vi "Insert General.vi"(6 "Time Stamp":timestamp, 8 "error in (no error)":errorcluster, 9 "Data":T1, 10 "Paths":T2, 11 "Data.PG in":refnum<class "Data.PG.lvclass">) -> (0 "error out":errorcluster, 3 "Data.PG out":refnum<class "Data.PG.lvclass">)   [LabVIEW 2020, in "Data.PG.lvclass"]
uses:
  Data.PG.lvclass
  Data/Typedefs/Operation--enum.ctl
  Data.PG.lvclass/Data.PG.ctl
  <vilib>/JDP Science/PostgreSQL Library/Result/PQ Result.lvclass/PQ Result.ctl
  <vilib>/JDP Science/PostgreSQL Library/Connection/Execute Command (2D string results).vi
  <vilib>/JDP Science/PostgreSQL Library/Result/Clear.vi
  <vilib>/JDP Science/PostgreSQL Library/Connection/Execute Command (Result).vi
  <vilib>/JDP Science/PostgreSQL Library/Connection/Execute (Return first result with rows).vi
  <vilib>/JDP Science/PostgreSQL Library/Connection/Single Command with parameters.vi
  <vilib>/JDP Science/PostgreSQL Library/Result/Get all results as 2D strings array.vi
  <vilib>/JDP Science/PostgreSQL Library/Connection/PQ Connection.lvclass
  Data/Data.lvclass
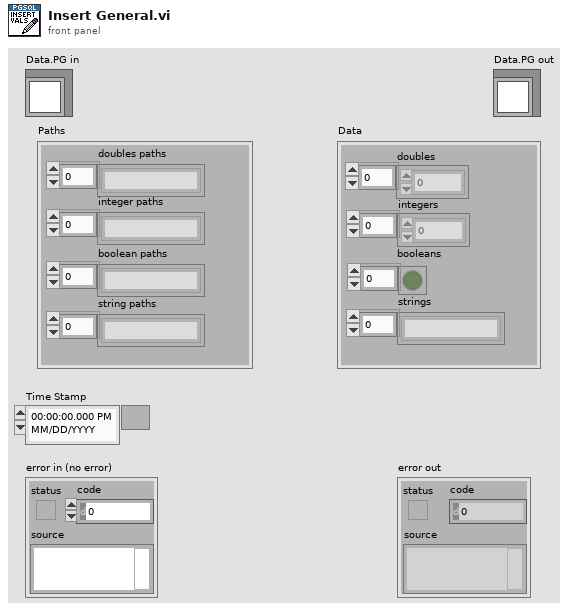
[diagram p1: front panel]
types:
  T1 = cluster{"doubles":dbl[], "integers":i32[], "booleans":bool[], "strings":string[]}
  T2 = cluster{"doubles paths":string[], "integer paths":string[], "boolean paths":string[], "string paths":string[]}
  T3 = typedef "Data.lvclass/Operation--enum.ctl" = enum16{"Read", "Write", "Write + Append"}
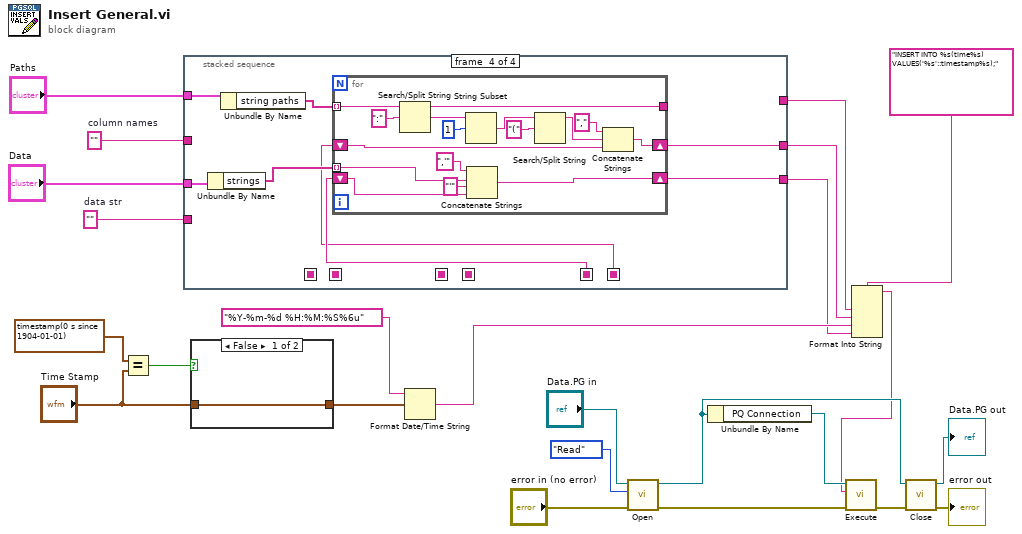
[diagram p0: block diagram]
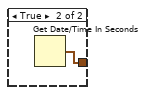
[diagram p2: hidden frame]
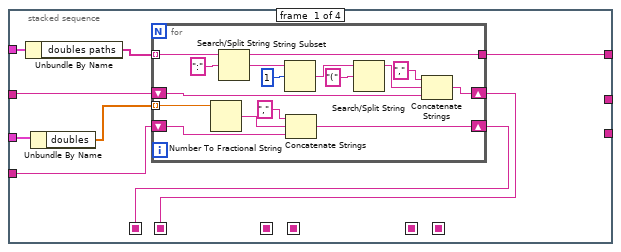
[diagram p3: hidden frame]
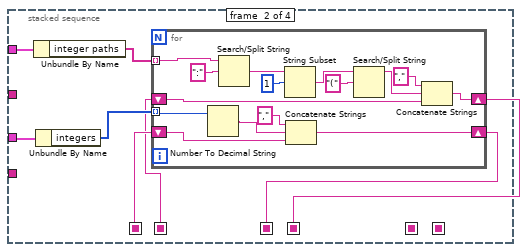
[diagram p4: hidden frame]
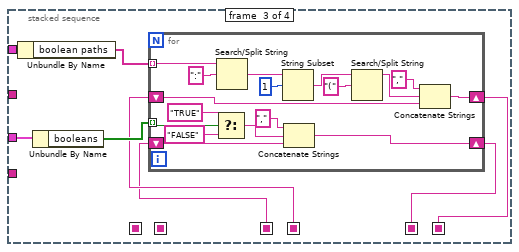
[diagram p5: hidden frame]
diagram:
  w21 = ""  # data str
  w22 = ""  # column names
  n1 = Equal?(x=timestamp(0 s since 1904-01-01), y="Time Stamp") -> (x = y?=w18:bool)
  n2 = stacked-sequence {
    seq-local: [w26 _ _ _] -> [_ w50 _ _]
    seq-local: [w25 _ _ _] -> [_ w54 _ _]
    seq-local: [_ w55 _ _] -> [_ _ w76 _]
    seq-local: [_ w51 _ _] -> [_ _ w75 _]
    seq-local: [_ _ w73 _] -> [_ _ _ w98]
    seq-local: [_ _ w74 _] -> [_ _ _ w99]
    tunnel: "Paths" -> [w33 w57 w79 w105]
    tunnel: "Data" -> [w32 w53 w80 w103]
    tunnel: w22 -> [w30 _ _ _]
    tunnel: w21 -> [w29 _ _ _]
    tunnel: [w27 _ _ _] -> w4
    tunnel: [_ _ _ w101] -> w3
    tunnel: [_ _ _ w100] -> w1
    frame #0 {
      n3 = Unbundle By Name(w33) -> ("doubles paths"=w31:string[])
      n4 = Unbundle By Name(w32) -> ("doubles"=w28:dbl[])
      n5 = for {
        tunnel: w31 -> [w46] mode=indexing
        tunnel: w28 -> [w41] mode=indexing
        shift-right: [w45] -> w26
        shift-left: w30 -> [w44]
        tunnel: [w43] -> w27
        shift-right: [w38] -> w25
        shift-left: w29 -> [w37]
        n6 = Number To Fractional String(number=w41) -> (F-format string=w40:string)  [unwired: 3 in]
        n7 = Search/Split String(string=w46, search string/char (-)=":") -> (substring before match=w43:string, match + rest of string=w48:string)  [unwired: 1 in, 1 out]
        n8 = String Subset(string=w48, offset (0)=1) -> (substring=w36:string)  [unwired: 1 in]
        n9 = Concatenate Strings("," ("string"), w40, w37) -> (w38:string)
        n10 = Search/Split String(string=w36, search string/char (-)="(") -> (substring before match=w35:string)  [unwired: 1 in, 2 out]
        n11 = Concatenate Strings("," ("string"), w35, w44) -> (w45:string)
      }
    }
    frame #1 {
      n12 = Unbundle By Name(w57) -> ("integer paths"=w56:string[])
      n13 = Unbundle By Name(w53) -> ("integers"=w52:i32[])
      n14 = for {
        tunnel: w56 -> [w60] mode=indexing
        tunnel: w52 -> [w58] mode=indexing
        shift-right: [w69] -> w55
        shift-left: w50 -> [w68]
        shift-right: [w65] -> w51
        shift-left: w54 -> [w64]
        n15 = Number To Decimal String(number=w58) -> (decimal integer string=w59:string)  [unwired: 1 in]
        n16 = Search/Split String(string=w60, search string/char (-)=":") -> (match + rest of string=w71:string)  [unwired: 1 in, 2 out]
        n17 = String Subset(string=w71, offset (0)=1) -> (substring=w63:string)  [unwired: 1 in]
        n18 = Concatenate Strings("," ("string"), w59, w64) -> (w65:string)
        n19 = Search/Split String(string=w63, search string/char (-)="(") -> (substring before match=w62:string)  [unwired: 1 in, 2 out]
        n20 = Concatenate Strings("," ("string"), w62, w68) -> (w69:string)
      }
    }
    frame #2 {
      n21 = Unbundle By Name(w79) -> ("boolean paths"=w78:string[])
      n22 = Unbundle By Name(w80) -> ("booleans"=w77:bool[])
      n23 = for {
        tunnel: w78 -> [w94] mode=indexing
        shift-right: [w93] -> w73
        shift-left: w76 -> [w92]
        shift-right: [w89] -> w74
        shift-left: w75 -> [w88]
        tunnel: w77 -> [w81] mode=indexing
        n24 = Select(t="TRUE", s=w81, f="FALSE") -> (s? t:f=w84:string)
        n25 = Search/Split String(string=w94, search string/char (-)=":") -> (match + rest of string=w96:string)  [unwired: 1 in, 2 out]
        n26 = String Subset(string=w96, offset (0)=1) -> (substring=w87:string)  [unwired: 1 in]
        n27 = Concatenate Strings("," ("string"), w84, w88) -> (w89:string)
        n28 = Search/Split String(string=w87, search string/char (-)="(") -> (substring before match=w86:string)  [unwired: 1 in, 2 out]
        n29 = Concatenate Strings("," ("string"), w86, w92) -> (w93:string)
      }
    }
    frame #3 {
      n30 = Unbundle By Name(w103) -> ("strings"=w102:string[])
      n31 = Unbundle By Name(w105) -> ("string paths"=w104:string[])
      n32 = for {
        tunnel: w104 -> [w118] mode=indexing
        shift-right: [w117] -> w101
        shift-left: w98 -> [w116]
        tunnel: [w115] -> _
        shift-right: [w112] -> w100
        shift-left: w99 -> [w107]
        tunnel: w102 -> [w108] mode=indexing
        n33 = Search/Split String(string=w118, search string/char (-)=":") -> (substring before match=w115:string, match + rest of string=w120:string)  [unwired: 1 in, 1 out]
        n34 = String Subset(string=w120, offset (0)=1) -> (substring=w111:string)  [unwired: 1 in]
        n35 = Concatenate Strings(",'" ("string"), w108, "'" ("string"), w107) -> (w112:string)
        n36 = Search/Split String(string=w111, search string/char (-)="(") -> (substring before match=w110:string)  [unwired: 1 in, 2 out]
        n37 = Concatenate Strings("," ("string"), w110, w116) -> (w117:string)
      }
    }
  }
  n38 = case shown="False" w18 {
    tunnel: [w122 w123] -> w19
    tunnel: "Time Stamp" -> [w122 _]
    frame False {
    }
    frame True {
      n39 = Get Date/Time In Seconds() -> (seconds since 1Jan1904=w123:timestamp)
    }
  }
  n40 = Format Date/Time String(time format string (%c)="%Y-%m-%d %H:%M:%S%6u", seconds (now)=w19) -> (date/time string=w2:string)  [unwired: 1 in]
  n41 = call-dynamic "Open.vi"("error in (no error)"="error in (no error)", "Operation"=Operation--enum."Read", "Data.PG in"="Data.PG in") -> ("error out"=w12:errorcluster, "Data.PG out"=w8:refnum<class "Data.PG.lvclass">)  [unwired: 7 in]
  n42 = Unbundle By Name(w8) -> ("PQ Connection"=w7:refnum<class "PQ Connection.lvclass">)
  n43 = Format Into String(format string="INSERT INTO %s(time%s) VALUES('%s'::timestamp%s);", w4, w3, w2, w1) -> (resulting string=w6:string)  [unwired: 2 in, 1 out]
  n44 = call-poly <vilib>:"Execute.vi"("error in (no error)"=w12, "SQL"=w6, "PQ Connection in"=w7) -> ("error out"=w11:errorcluster)  [unwired: 5 in, 3 out]
  n45 = call-dynamic "Close.vi"("error in (no error)"=w11, "Data.PG in"=w8) -> ("error out"=→"error out":errorcluster, "Data.PG out"=→"Data.PG out":refnum<class "Data.PG.lvclass">)  [unwired: 8 in]
